vi "GEOM_SaveReqROI.vi"(9 "clean":bool, 10 "GEOM_RequestedROI":T1) -> (2 "ROIs out":T1[](array[typedef]))   [LabVIEW 2016]
uses:
  GEOM_Coords.ctl
  GEOM_VAR_action.ctl
  GEOM_Gbls.vi
  DBSHAND/private/vis/DatabaseHand_Element_Set(string).vi
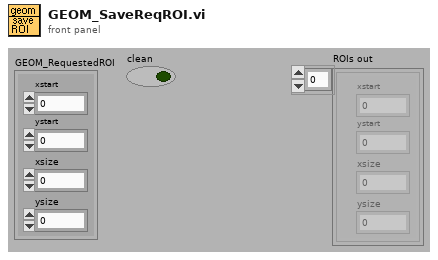
[diagram p1: front panel]
types:
  T1 = typedef "GEOM_Coords.ctl" = cluster{"xstart":u32, "ystart":u32, "xsize":u32, "ysize":u32}
  T2 = typedef "GEOM_VAR_action.ctl" = enum16{"read", "write"}
  T3 = typedef "DatabaseHand_RefNum.ctl" = refnum<vi>
  T4 = cluster{"xstart":i32, "ystart":i32, "xsize":i32, "ysize":i32}[]
  T5 = cluster{"xstart":i32, "ystart":i32, "xsize":i32, "ysize":i32}
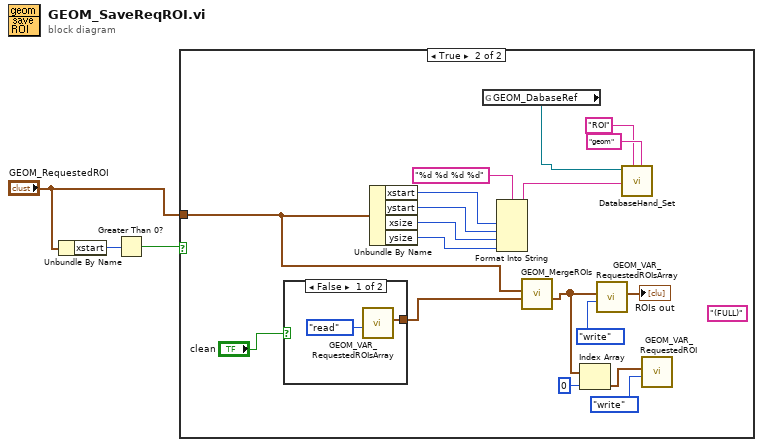
[diagram p0: block diagram]
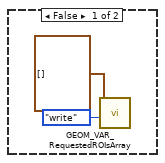
[diagram p2: hidden frame]
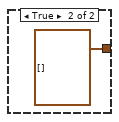
[diagram p3: hidden frame]
diagram:
  n1 = Unbundle By Name("GEOM_RequestedROI") -> ("xstart"=w2:u32)
  n2 = Greater Than 0?(x=w2) -> (x > 0?=w1:bool)
  n3 = case shown="True" w1 {
    tunnel: "GEOM_RequestedROI" -> [_ w9]
    frame False {
      n4 = call "GEOM_VAR_RequestedROIsArray.vi"("Action"=GEOM_VAR_action."write", "ROIs"=T1[] []) -> ()  [unwired: 10 out]
    }
    frame True {
      (unwired) "(FULL)"
      n5 = case shown="False" "clean" {
        tunnel: [w24 T1[] [] ("ROIs out")] -> w13
        frame False {
          n6 = call "GEOM_VAR_RequestedROIsArray.vi"("Action"=GEOM_VAR_action."read") -> ("ROIs out"=w24:T1[])  [unwired: 1 in, 9 out]
        }
        frame True {
        }
      }
      n7 = Unbundle By Name(w9) -> ("xstart"=w20:u32, "ystart"=w19:u32, "xsize"=w18:u32, "ysize"=w17:u32)
      n8 = global read "GEOM_Gbls.vi" "GEOM_DabaseRef"() -> (w15:T3)
      n9 = Format Into String(format string="%d %d %d %d", w20, w19, w18, w17) -> (resulting string=w16:string)  [unwired: 2 in, 1 out]
      n10 = call "GEOM_MergeROIs.vi"("curr rois"=w13, "new roi"=w9) -> ("rois out"=w8:T4)  [unwired: 9 out]
      n11 = Index Array(array=w8, index=0) -> (element=w6:T5)
      n12 = call "GEOM_VAR_RequestedROIsArray.vi"("Action"=GEOM_VAR_action."write", "ROIs"=w8) -> ("ROIs out"=→"ROIs out":T1[])  [unwired: 9 out]
      n13 = call-poly "DatabaseHand_Set.vi"("group"="geom", "name"="ROI", "value"=w16, "Database RefNum in"=w15) -> ()  [unwired: 4 in, 4 out]
      n14 = call "GEOM_VAR_RequestedROI.vi"("Action"=GEOM_VAR_action."write", "GEOM_RequestedROI"=w6) -> ()  [unwired: 10 out]
    }
  }
